vi "Control_Panel_Globals.vi"() -> ()   [LabVIEW 2019]
uses:
  Control_Panel_Cluster.ctl
  Control_Panel_States.ctl
panel:
  in  "Control_Panel_State":T1
  in  "Control_Panel_Output":dbl
  in  "Control_Panel_Motor":string="Control_Panel_Motor"
  in  "Control_Panel_Execute_Notifier":refnum<notifier>
  in  "Control_Panel_Set_Notifier":refnum<notifier>
  in  "Control_Panel_Execute_Ref":string="Control_Panel_Execute_Ref"
  in  "Control_Panel_Set_Ref":string="Control_Panel_Set_Ref"
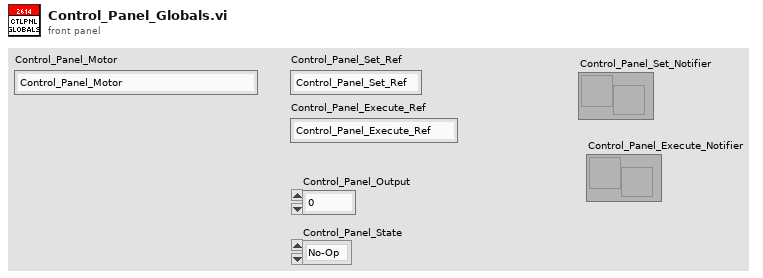
[diagram p1: front panel]
types:
  T1 = typedef "Control_Panel_States.ctl" = enum16{"No-Op", "Rotational_Control", "Positional_Control", "Manual_Control"}
diagram:
